vi "GeoData.vi"() -> ()   [LabVIEW 2017] (continued)
UT\tCache County\tH1\n84318\t49005\tHyde park\tUT\tCache County\tH1\n84338\t49005\tTrenton\tUT\tCache County\tH1\n84332\t49005\tProvidence\tUT\tCache County\tH1\n84305\t49005\tClarkston\tUT\tCache County\tH1\n84312\t49005\tGarland\tUT\tCache County\tH1\n84328\t49005\tParadise\tUT\tCache County\tH1\n84341\t49005\tLogan\tUT\tCache County\tH1\n84322\t49005\tLogan\tUT\tCache County\tH1\n84319\t49005\tHyrum\tUT\tCache County\tH1\n84325\t49005\tMendon\tUT\tCache County\tH1\n84320\t49005\tLewiston\tUT\tCache County\tH1\n84501\t49007\tPrice\tUT\tCarbon County\tH1\n84529\t49007\tKenilworth\tUT\tCarbon County\tH1\n84542\t49007\tWellington\tUT\tCarbon County\tH1\n84526\t49007\tHelper\tUT\tCarbon County\tH1\n84520\t49007\tEast carbon\tUT\tCarbon County\tH1\n84539\t49007\tSunnyside\tUT\tCarbon County\tH1\n84046\t49009\tManila\tUT\tDaggett County\tH1\n84023\t49009\tDutch john\tUT\tDaggett County\tH1\n84054\t49011\tNorth salt lake\tUT\tDavis County\tH1\n84315\t49011\tHooper\tUT\tDavis County\tH1\n84011\t49011\tBountiful\tUT\tDavis County\tH1\n84075\t49011\tSyracuse\tUT\tDavis County\tH1\n84041\t49011\tLayton\tUT\tDavis County\tH1\n84037\t49011\tKaysville\tUT\tDavis County\tH1\n84405\t49011\tOgden\tUT\tDavis County\tH1\n84025\t49011\tFarmington\tUT\tDavis County\tH1\n84014\t49011\tCenterville\tUT\tDavis County\tH1\n84015\t49011\tClearfield\tUT\tDavis County\tH1\n84087\t49011\tWoods cross\tUT\tDavis County\tH1\n84016\t49011\tClearfield\tUT\tDavis County\tH1\n84089\t49011\tClearfield\tUT\tDavis County\tH1\n84010\t49011\tBountiful\tUT\tDavis County\tH1\n84040\t49011\tLayton\tUT\tDavis County\tH1\n84056\t49011\tHill afb\tUT\tDavis County\tH1\n84031\t49013\tHanna\tUT\tDuchesne County\tH1\n84066\t49013\tRoosevelt\tUT\tDuchesne County\tH1\n84072\t49013\tTabiona\tUT\tDuchesne County\tH1\n84073\t49013\tTalmage\tUT\tDuchesne County\tH1\n84052\t49013\tMyton\tUT\tDuchesne County\tH1\n84021\t49013\tDuchesne\tUT\tDuchesne County\tH1\n84051\t49013\tMountain home\tUT\tDuchesne County\tH1\n84007\t49013\tBluebell\tUT\tDuchesne County\tH1\n84053\t49013\tNeola\tUT\tDuchesne County\tH1\n84001\t49013\tAltamont\tUT\tDuchesne County\tH1\n84002\t49013\tAltonah\tUT\tDuchesne County\tH1\n84027\t49013\tFruitland\tUT\tDuchesne County\tH1\n84501\t49015\tPrice\tUT\tEmery County\tH1\n84521\t49015\tElmo\tUT\tEmery County\tH1\n84523\t49015\tFerron\tUT\tEmery County\tH1\n84537\t49015\tOrangeville\tUT\tEmery County\tH1\n84522\t49015\tEmery\tUT\tEmery County\tH1\n84518\t49015\tCleveland\tUT\tEmery County\tH1\n84528\t49015\tHuntington\tUT\tEmery County\tH1\n84525\t49015\tGreen river\tUT\tEmery County\tH1\n84516\t49015\tClawson\tUT\tEmery County\tH1\n84513\t49015\tCastle dale\tUT\tEmery County\tH1\n84716\t49017\tBoulder\tUT\tGarfield County\tH1\n84718\t49017\tCannonville\tUT\tGarfield County\tH1\n84764\t49017\tBryce\tUT\tGarfield County\tH1\n84736\t49017\tHenrieville\tUT\tGarfield County\tH1\n84712\t49017\tAntimony\tUT\tGarfield County\tH1\n84726\t49017\tEscalante\tUT\tGarfield County\tH1\n84759\t49017\tPanguitch\tUT\tGarfield County\tH1\n84776\t49017\tTropic\tUT\tGarfield County\tH1\n84515\t49019\tCisco\tUT\tGrand County\tH1\n84525\t49019\tGreen river\tUT\tGrand County\tH1\n84532\t49019\tMoab\tUT\tGrand County\tH1\n84540\t49019\tThompson\tUT\tGrand County\tH1\n84781\t49021\tPine valley\tUT\tIron County\tH1\n84722\t49021\tCentral\tUT\tIron County\tH1\n84761\t49021\tParowan\tUT\tIron County\tH1\n84721\t49021\tCedar city\tUT\tIron County\tH1\n84720\t49021\tCedar city\tUT\tIron County\tH1\n84742\t49021\tKanarraville\tUT\tIron County\tH1\n84757\t49021\tNew harmony\tUT\tIron County\tH1\n84714\t49021\tBeryl\tUT\tIron County\tH1\n84753\t49021\tModena\tUT\tIron County\tH1\n84719\t49021\tBrian head\tUT\tIron County\tH1\n84756\t49021\tNewcastle\tUT\tIron County\tH1\n84760\t49021\tParagonah\tUT\tIron County\tH1\n84737\t49021\tHurricane\tUT\tIron County\tH1\n84772\t49021\tSummit\tUT\tIron County\tH1\n84639\t49023\tLevan\tUT\tJuab County\tH1\n84628\t49023\tEureka\tUT\tJuab County\tH1\n84648\t49023\tNephi\tUT\tJuab County\tH1\n84645\t49023\tMona\tUT\tJuab County\tH1\n84758\t49025\tOrderville\tUT\tKane County\tH1\n84735\t49025\tHatch\tUT\tKane County\tH1\n84729\t49025\tGlendale\tUT\tKane County\tH1\n84710\t49025\tAlton\tUT\tKane County\tH1\n84726\t49025\tEscalante\tUT\tKane County\tH1\n84762\t49025\tDuck creek village\tUT\tKane County\tH1\n84755\t49025\tMount carmel\tUT\tKane County\tH1\n84741\t49025\tKanab\tUT\tKane County\tH1\n84635\t49027\tHinckley\tUT\tMillard County\tH1\n84656\t49027\tScipio\tUT\tMillard County\tH1\n84631\t49027\tFillmore\tUT\tMillard County\tH1\n84640\t49027\tLynndyl\tUT\tMillard County\tH1\n84728\t49027\tGarrison\tUT\tMillard County\tH1\n84649\t49027\tOak city\tUT\tMillard County\tH1\n84638\t49027\tLeamington\tUT\tMillard County\tH1\n84637\t49027\tKanosh\tUT\tMillard County\tH1\n84624\t49027\tDelta\tUT\tMillard County\tH1\n84636\t49027\tHolden\tUT\tMillard County\tH1\n84644\t49027\tMeadow\tUT\tMillard County\tH1\n84018\t49029\tCroydon\tUT\tMorgan County\tH1\n84050\t49029\tMorgan\tUT\tMorgan County\tH1\n84017\t49029\tCoalville\tUT\tMorgan County\tH1\n84750\t49031\tMarysvale\tUT\tPiute County\tH1\n84743\t49031\tKingston\tUT\tPiute County\tH1\n84712\t49031\tAntimony\tUT\tPiute County\tH1\n84732\t49031\tGreenwich\tUT\tPiute County\tH1\n84723\t49031\tCircleville\tUT\tPiute County\tH1\n84740\t49031\tJunction\tUT\tPiute County\tH1\n84064\t49033\tRandolph\tUT\tRich County\tH1\n84086\t49033\tWoodruff\tUT\tRich County\tH1\n84038\t49033\tLaketown\tUT\tRich County\tH1\n84028\t49033\tGarden city\tUT\tRich County\tH1\n84070\t49035\tSandy\tUT\tSalt Lake County\tH1\n84123\t49035\tSalt lake city\tUT\tSalt Lake County\tH1\n84129\t49035\tSalt lake city\tUT\tSalt Lake County\tH1\n84152\t49035\tSalt lake city\tUT\tSalt Lake County\tH1\n84101\t49035\tSalt lake city\tUT\tSalt Lake County\tH1\n84103\t49035\tSalt lake city\tUT\tSalt Lake County\tH1\n84118\t49035\tSalt lake city\tUT\tSalt Lake County\tH1\n84127\t49035\tSalt lake city\tUT\tSalt Lake County\tH1\n84134\t49035\tSalt lake city\tUT\tSalt Lake County\tH1\n84184\t49035\tSalt lake city\tUT\tSalt Lake County\tH1\n84119\t49035\tWest valley city\tUT\tSalt Lake County\tH1\n84138\t49035\tSalt lake city\tUT\tSalt Lake County\tH1\n84143\t49035\tSalt lake city\tUT\tSalt Lake County\tH1\n84047\t49035\tMidvale\tUT\tSalt Lake County\tH1\n84050\t49035\tMorgan\tUT\tSalt Lake County\tH1\n84107\t49035\tSalt lake city\tUT\tSalt Lake County\tH1\n84092\t49035\tSandy\tUT\tSalt Lake County\tH1\n84158\t49035\tSalt lake city\tUT\tSalt Lake County\tH1\n84112\t49035\tSalt lake city\tUT\tSalt Lake County\tH1\n84132\t49035\tSalt lake city\tUT\tSalt Lake County\tH1\n84009\t49035\tSouth jordan\tUT\tSalt Lake County\tH1\n84065\t49035\tRiverton\tUT\tSalt Lake County\tH1\n84084\t49035\tWest jordan\tUT\tSalt Lake County\tH1\n84102\t49035\tSalt lake city\tUT\tSalt Lake County\tH1\n84106\t49035\tSalt lake city\tUT\tSalt Lake County\tH1\n84115\t49035\tSalt lake city\tUT\tSalt Lake County\tH1\n84090\t49035\tSandy\tUT\tSalt Lake County\tH1\n84096\t49035\tHerriman\tUT\tSalt Lake County\tH1\n84088\t49035\tWest jordan\tUT\tSalt Lake County\tH1\n84105\t49035\tSalt lake city\tUT\tSalt Lake County\tH1\n84150\t49035\tSalt lake city\tUT\tSalt Lake County\tH1\n84122\t49035\tSalt lake city\tUT\tSalt Lake County\tH1\n84141\t49035\tSalt lake city\tUT\tSalt Lake County\tH1\n84139\t49035\tSalt lake city\tUT\tSalt Lake County\tH1\n84020\t49035\tDraper\tUT\tSalt Lake County\tH1\n84157\t49035\tSalt lake city\tUT\tSalt Lake County\tH1\n84104\t49035\tSalt lake city\tUT\tSalt Lake County\tH1\n84120\t49035\tWest valley city\tUT\tSalt Lake County\tH1\n84121\t49035\tSalt lake city\tUT\tSalt Lake County\tH1\n84133\t49035\tSalt lake city\tUT\tSalt Lake County\tH1\n84113\t49035\tSalt lake city\tUT\tSalt Lake County\tH1\n84148\t49035\tSalt lake city\tUT\tSalt Lake County\tH1\n84128\t49035\tWest valley city\tUT\tSalt Lake County\tH1\n84108\t49035\tSalt lake city\tUT\tSalt Lake County\tH1\n84117\t49035\tSalt lake city\tUT\tSalt Lake County\tH1\n84095\t49035\tSouth jordan\tUT\tSalt Lake County\tH1\n84093\t49035\tSandy\tUT\tSalt Lake County\tH1\n84126\t49035\tSalt lake city\tUT\tSalt Lake County\tH1\n84165\t49035\tSalt lake city\tUT\tSalt Lake County\tH1\n84171\t49035\tSalt lake city\tUT\tSalt Lake County\tH1\n84110\t49035\tSalt lake city\tUT\tSalt Lake County\tH1\n84091\t49035\tSandy\tUT\tSalt Lake County\tH1\n84199\t49035\tSalt lake city\tUT\tSalt Lake County\tH1\n84190\t49035\tSalt lake city\tUT\tSalt Lake County\tH1\n84151\t49035\tSalt lake city\tUT\tSalt Lake County\tH1\n84124\t49035\tSalt lake city\tUT\tSalt Lake County\tH1\n84109\t49035\tSalt lake city\tUT\tSalt Lake County\tH1\n84094\t49035\tSandy\tUT\tSalt Lake County\tH1\n84116\t49035\tSalt lake city\tUT\tSalt Lake County\tH1\n84125\t49035\tSalt lake city\tUT\tSalt Lake County\tH1\n84044\t49035\tMagna\tUT\tSalt Lake County\tH1\n84081\t49035\tWest jordan\tUT\tSalt Lake County\tH1\n84111\t49035\tSalt lake city\tUT\tSalt Lake County\tH1\n84180\t49035\tSalt lake city\tUT\tSalt Lake County\tH1\n84006\t49035\tBingham canyon\tUT\tSalt Lake County\tH1\n84170\t49035\tSalt lake city\tUT\tSalt Lake County\tH1\n84114\t49035\tSalt lake city\tUT\tSalt Lake County\tH1\n84533\t49037\tLake powell\tUT\tSan Juan County\tH1\n84512\t49037\tBluff\tUT\tSan Juan County\tH1\n84511\t49037\tBlanding\tUT\tSan Juan County\tH1\n84535\t49037\tMonticello\tUT\tSan Juan County\tH1\n84531\t49037\tMexican hat\tUT\tSan Juan County\tH1\n84532\t49037\tMoab\tUT\tSan Juan County\tH1\n84510\t49037\tAneth\tUT\tSan Juan County\tH1\n84530\t49037\tLa sal\tUT\tSan Juan County\tH1\n84534\t49037\tMontezuma creek\tUT\tSan Juan County\tH1\n84536\t49037\tMonument valley\tUT\tSan Juan County\tH1\n84629\t49039\tFairview\tUT\tSanpete County\tH1\n84622\t49039\tCenterfield\tUT\tSanpete County\tH1\n84630\t49039\tFayette\tUT\tSanpete County\tH1\n84665\t49039\tSterling\tUT\tSanpete County\tH1\n84647\t49039\tMount pleasant\tUT\tSanpete County\tH1\n84627\t49039\tEphraim\tUT\tSanpete County\tH1\n84642\t49039\tManti\tUT\tSanpete County\tH1\n84667\t49039\tWales\tUT\tSanpete County\tH1\n84643\t49039\tMayfield\tUT\tSanpete County\tH1\n84634\t49039\tGunnison\tUT\tSanpete County\tH1\n84632\t49039\tFountain green\tUT\tSanpete County\tH1\n84621\t49039\tAxtell\tUT\tSanpete County\tH1\n84662\t49039\tSpring city\tUT\tSanpete County\tH1\n84646\t49039\tMoroni\tUT\tSanpete County\tH1\n84623\t49039\tChester\tUT\tSanpete County\tH1\n84739\t49041\tJoseph\tUT\tSevier County\tH1\n84754\t49041\tMonroe\tUT\tSevier County\tH1\n84654\t49041\tSalina\tUT\tSevier County\tH1\n84620\t49041\tAurora\tUT\tSevier County\tH1\n84744\t49041\tKoosharem\tUT\tSevier County\tH1\n84711\t49041\tAnnabella\tUT\tSevier County\tH1\n84730\t49041\tGlenwood\tUT\tSevier County\tH1\n84657\t49041\tSigurd\tUT\tSevier County\tH1\n84701\t49041\tRichfield\tUT\tSevier County\tH1\n84766\t49041\tSevier\tUT\tSevier County\tH1\n84652\t49041\tRedmond\tUT\tSevier County\tH1\n84724\t49041\tElsinore\tUT\tSevier County\tH1\n84033\t49043\tHenefer\tUT\tSummit County\tH1\n84024\t49043\tEcho\tUT\tSummit County\tH1\n84055\t49043\tOakley\tUT\tSummit County\tH1\n84060\t49043\tPark city\tUT\tSummit County\tH1\n84017\t49043\tCoalville\tUT\tSummit County\tH1\n84036\t49043\tKamas\tUT\tSummit County\tH1\n84068\t49043\tPark city\tUT\tSummit County\tH1\n84098\t49043\tPark city\tUT\tSummit County\tH1\n84061\t49043\tPeoa\tUT\tSummit County\tH1\n84074\t49045\tTooele\tUT\tTooele County\tH1\n84029\t49045\tGrantsville\tUT\tTooele County\tH1\n84034\t49045\tIbapah\tUT\tTooele County\tH1\n84083\t49045\tWendover\tUT\tTooele County\tH1\n84069\t49045\tRush valley\tUT\tTooele County\tH1\n84071\t49045\tStockton\tUT\tTooele County\tH1\n84022\t49045\tDugway\tUT\tTooele County\tH1\n84080\t49045\tVernon\tUT\tTooele County\tH1\n84079\t49047\tVernal\tUT\tUintah County\tH1\n84066\t49047\tRoosevelt\tUT\tUintah County\tH1\n84035\t49047\tJensen\tUT\tUintah County\tH1\n84063\t49047\tRandlett\tUT\tUintah County\tH1\n84078\t49047\tVernal\tUT\tUintah County\tH1\n84039\t49047\tLapoint\tUT\tUintah County\tH1\n84026\t49047\tFort duchesne\tUT\tUintah County\tH1\n84085\t49047\tWhiterocks\tUT\tUintah County\tH1\n84076\t49047\tTridell\tUT\tUintah County\tH1\n84008\t49047\tBonanza\tUT\tUintah County\tH1\n84043\t49049\tLehi\tUT\tUtah County\tH1\n84059\t49049\tOrem\tUT\tUtah County\tH1\n84004\t49049\tAlpine\tUT\tUtah County\tH1\n84097\t49049\tOrem\tUT\tUtah County\tH1\n84013\t49049\tCedar valley\tUT\tUtah County\tH1\n84603\t49049\tProvo\tUT\tUtah County\tH1\n84604\t49049\tProvo\tUT\tUtah County\tH1\n84655\t49049\tSantaquin\tUT\tUtah County\tH1\n84032\t49049\tHeber city\tUT\tUtah County\tH1\n84602\t49049\tProvo\tUT\tUtah County\tH1\n84005\t49049\tEagle mountain\tUT\tUtah County\tH1\n84020\t49049\tDraper\tUT\tUtah County\tH1\n84062\t49049\tPleasant grove\tUT\tUtah County\tH1\n84058\t49049\tOrem\tUT\tUtah County\tH1\n84660\t49049\tSpanish fork\tUT\tUtah County\tH1\n84606\t49049\tProvo\tUT\tUtah County\tH1\n84003\t49049\tAmerican fork\tUT\tUtah County\tH1\n84601\t49049\tProvo\tUT\tUtah County\tH1\n84651\t49049\tPayson\tUT\tUtah County\tH1\n84605\t49049\tProvo\tUT\tUtah County\tH1\n84626\t49049\tElberta\tUT\tUtah County\tH1\n84057\t49049\tOrem\tUT\tUtah County\tH1\n84045\t49049\tSaratoga springs\tUT\tUtah County\tH1\n84042\t49049\tLindon\tUT\tUtah County\tH1\n84663\t49049\tSpringville\tUT\tUtah County\tH1\n84653\t49049\tSalem\tUT\tUtah County\tH1\n84664\t49049\tMapleton\tUT\tUtah County\tH1\n84633\t49049\tGoshen\tUT\tUtah County\tH1\n84604\t49051\tProvo\tUT\tWasatch County\tH1\n84082\t49051\tWallsburg\tUT\tWasatch County\tH1\n84032\t49051\tHeber city\tUT\tWasatch County\tH1\n84060\t49051\tPark city\tUT\tWasatch County\tH1\n84036\t49051\tKamas\tUT\tWasatch County\tH1\n84049\t49051\tMidway\tUT\tWasatch County\tH1\n84779\t49053\tVirgin\tUT\tWashington County\tH1\n84781\t49053\tPine valley\tUT\tWashington County\tH1\n84763\t49053\tRockville\tUT\tWashington County\tH1\n84722\t49053\tCentral\tUT\tWashington County\tH1\n84733\t49053\tGunlock\tUT\tWashington County\tH1\n84782\t49053\tVeyo\tUT\tWashington County\tH1\n84784\t49053\tHildale\tUT\tWashington County\tH1\n84780\t49053\tWashington\tUT\tWashington County\tH1\n84791\t49053\tSaint george\tUT\tWashington County\tH1\n84720\t49053\tCedar city\tUT\tWashington County\tH1\n84765\t49053\tSanta clara\tUT\tWashington County\tH1\n84771\t49053\tSaint george\tUT\tWashington County\tH1\n84783\t49053\tDammeron valley\tUT\tWashington County\tH1\n84757\t49053\tNew harmony\tUT\tWashington County\tH1\n84790\t49053\tSaint george\tUT\tWashington County\tH1\n84745\t49053\tLa verkin\tUT\tWashington County\tH1\n84746\t49053\tLeeds\tUT\tWashington County\tH1\n84738\t49053\tIvins\tUT\tWashington County\tH1\n84774\t49053\tToquerville\tUT\tWashington County\tH1\n84767\t49053\tSpringdale\tUT\tWashington County\tH1\n84725\t49053\tEnterprise\tUT\tWashington County\tH1\n84770\t49053\tSaint george\tUT\tWashington County\tH1\n84737\t49053\tHurricane\tUT\tWashington County\tH1\n84715\t49055\tBicknell\tUT\tWayne County\tH1\n84734\t49055\tHanksville\tUT\tWayne County\tH1\n84747\t49055\tLoa\tUT\tWayne County\tH1\n84775\t49055\tTorrey\tUT\tWayne County\tH1\n84749\t49055\tLyman\tUT\tWayne County\tH1\n84773\t49055\tTeasdale\tUT\tWayne County\tH1\n84310\t49057\tEden\tUT\tWeber County\tH1\n84315\t49057\tHooper\tUT\tWeber County\tH1\n84407\t49057\tOgden\tUT\tWeber County\tH1\n84409\t49057\tOgden\tUT\tWeber County\tH1\n84201\t49057\tOgden\tUT\tWeber County\tH1\n84404\t49057\tOgden\tUT\tWeber County\tH1\n84405\t49057\tOgden\tUT\tWeber County\tH1\n84317\t49057\tHuntsville\tUT\tWeber County\tH1\n84415\t49057\tOgden\tUT\tWeber County\tH1\n84403\t49057\tOgden\tUT\tWeber County\tH1\n84414\t49057\tOgden\tUT\tWeber County\tH1\n84408\t49057\tOgden\tUT\tWeber County\tH1\n84402\t49057\tOgden\tUT\tWeber County\tH1\n84401\t49057\tOgden\tUT\tWeber County\tH1\n84067\t49057\tRoy\tUT\tWeber County\tH1\n84056\t49057\tHill afb\tUT\tWeber County\tH1\n84412\t49057\tOgden\tUT\tWeber County\tH1\n5733\t50001\tBrandon\tVT\tAddison County\tH1\n5747\t50001\tGranville\tVT\tAddison County\tH1\n5753\t50001\tMiddlebury\tVT\tAddison County\tH1\n5472\t50001\tNew haven\tVT\tAddison County\tH1\n5769\t50001\tSalisbury\tVT\tAddison County\tH1\n5469\t50001\tMonkton\tVT\tAddison County\tH1\n5748\t50001\tHancock\tVT\tAddison County\tH1\n5734\t50001\tBridport\tVT\tAddison County\tH1\n5770\t50001\tShoreham\tVT\tAddison County\tH1\n5766\t50001\tRipton\tVT\tAddison County\tH1\n5443\t50001\tBristol\tVT\tAddison County\tH1\n5456\t50001\tFerrisburgh\tVT\tAddison County\tH1\n5491\t50001\tVergennes\tVT\tAddison County\tH1\n5669\t50001\tRoxbury\tVT\tAddison County\tH1\n5740\t50001\tEast middlebury\tVT\tAddison County\tH1\n5461\t50001\tHinesburg\tVT\tAddison County\tH1\n5473\t50001\tNorth ferrisburgh\tVT\tAddison County\tH1\n5462\t50001\tHuntington\tVT\tAddison County\tH1\n5445\t50001\tCharlotte\tVT\tAddison County\tH1\n5487\t50001\tStarksboro\tVT\tAddison County\tH1\n5767\t50001\tRochester\tVT\tAddison County\tH1\n5760\t50001\tOrwell\tVT\tAddison County\tH1\n5778\t50001\tWhiting\tVT\tAddison County\tH1\n5255\t50003\tManchester center\tVT\tBennington County\tH1\n5340\t50003\tBondville\tVT\tBennington County\tH1\n5148\t50003\tLondonderry\tVT\tBennington County\tH1\n5261\t50003\tPownal\tVT\tBennington County\tH1\n5352\t50003\tStamford\tVT\tBennington County\tH1\n5343\t50003\tJamaica\tVT\tBennington County\tH1\n5775\t50003\tWest pawlet\tVT\tBennington County\tH1\n5155\t50003\tSouth londonderry\tVT\tBennington County\tH1\n5201\t50003\tBennington\tVT\tBennington County\tH1\n5250\t50003\tArlington\tVT\tBennington County\tH1\n5257\t50003\tNorth bennington\tVT\tBennington County\tH1\n5761\t50003\tPawlet\tVT\tBennington County\tH1\n5152\t50003\tPeru\tVT\tBennington County\tH1\n5252\t50003\tEast arlington\tVT\tBennington County\tH1\n5253\t50003\tEast dorset\tVT\tBennington County\tH1\n5262\t50003\tShaftsbury\tVT\tBennington County\tH1\n5254\t50003\tManchester\tVT\tBennington County\tH1\n5251\t50003\tDorset\tVT\tBennington County\tH1\n5768\t50003\tRupert\tVT\tBennington County\tH1\n5260\t50003\tNorth pownal\tVT\tBennington County\tH1\n5161\t50003\tWeston\tVT\tBennington County\tH1\n5363\t50003\tWilmington\tVT\tBennington County\tH1\n5350\t50003\tReadsboro\tVT\tBennington County\tH1\n5776\t50003\tWest rupert\tVT\tBennington County\tH1\n5680\t50005\tWolcott\tVT\tCaledonia County\tH1\n5839\t50005\tGlover\tVT\tCaledonia County\tH1\n5849\t50005\tLyndon\tVT\tCaledonia County\tH1\n5861\t50005\tPassumpsic\tVT\tCaledonia County\tH1\n5821\t50005\tBarnet\tVT\tCaledonia County\tH1\n5850\t50005\tLyndon center\tVT\tCaledonia County\tH1\n5832\t50005\tEast burke\tVT\tCaledonia County\tH1\n5873\t50005\tWest danville\tVT\tCaledonia County\tH1\n5647\t50005\tCabot\tVT\tCaledonia County\tH1\n5819\t50005\tSaint johnsbury\tVT\tCaledonia County\tH1\n5866\t50005\tSheffield\tVT\tCaledonia County\tH1\n5871\t50005\tWest burke\tVT\tCaledonia County\tH1\n5838\t50005\tEast saint johnsbury\tVT\tCaledonia County\tH1\n5081\t50005\tWells river\tVT\tCaledonia County\tH1\n5046\t50005\tGroton\tVT\tCaledonia County\tH1\n5836\t50005\tEast hardwick\tVT\tCaledonia County\tH1\n5837\t50005\tEast haven\tVT\tCaledonia County\tH1\n5862\t50005\tPeacham\tVT\tCaledonia County\tH1\n5828\t50005\tDanville\tVT\tCaledonia County\tH1\n5824\t50005\tConcord\tVT\tCaledonia County\tH1\n5867\t50005\tSutton\tVT\tCaledonia County\tH1\n5863\t50005\tSaint johnsbury center\tVT\tCaledonia County\tH1\n5842\t50005\tGreensboro bend\tVT\tCaledonia County\tH1\n5050\t50005\tMc indoe falls\tVT\tCaledonia County\tH1\n5069\t50005\tSouth ryegate\tVT\tCaledonia County\tH1\n5658\t50005\tMarshfield\tVT\tCaledonia County\tH1\n5841\t50005\tGreensboro\tVT\tCaledonia County\tH1\n5851\t50005\tLyndonville\tVT\tCaledonia County\tH1\n5843\t50005\tHardwick\tVT\tCaledonia County\tH1\n5042\t50005\tEast ryegate\tVT\tCaledonia County\tH1\n5848\t50005\tLower waterford\tVT\tCaledonia County\tH1\n5403\t50007\tSouth burlington\tVT\tChittenden County\tH1\n5446\t50007\tColchester\tVT\tChittenden County\tH1\n5449\t50007\tColchester\tVT\tChittenden County\tH1\n5676\t50007\tWaterbury\tVT\tChittenden County\tH1\n5490\t50007\tUnderhill center\tVT\tChittenden County\tH1\n5495\t50007\tWilliston\tVT\tChittenden County\tH1\n5401\t50007\tBurlington\tVT\tChittenden County\tH1\n5452\t50007\tEssex junction\tVT\tChittenden County\tH1\n5482\t50007\tShelburne\tVT\tChittenden County\tH1\n5406\t50007\tBurlington\tVT\tChittenden County\tH1\n5466\t50007\tJonesville\tVT\tChittenden County\tH1\n5402\t50007\tBurlington\tVT\tChittenden County\tH1\n5477\t50007\tRichmond\tVT\tChittenden County\tH1\n5465\t50007\tJericho\tVT\tChittenden County\tH1\n5453\t50007\tEssex junction\tVT\tChittenden County\tH1\n5451\t50007\tEssex\tVT\tChittenden County\tH1\n5439\t50007\tColchester\tVT\tChittenden County\tH1\n5408\t50007\tBurlington\tVT\tChittenden County\tH1\n5489\t50007\tUnderhill\tVT\tChittenden County\tH1\n5404\t50007\tWinooski\tVT\tChittenden County\tH1\n5468\t50007\tMilton\tVT\tChittenden County\tH1\n5478\t50007\tSaint albans\tVT\tChittenden County\tH1\n5454\t50007\tFairfax\tVT\tChittenden County\tH1\n5461\t50007\tHinesburg\tVT\tChittenden County\tH1\n5473\t50007\tNorth ferrisburgh\tVT\tChittenden County\tH1\n5462\t50007\tHuntington\tVT\tChittenden County\tH1\n5445\t50007\tCharlotte\tVT\tChittenden County\tH1\n5487\t50007\tStarksboro\tVT\tChittenden County\tH1\n5405\t50007\tBurlington\tVT\tChittenden County\tH1\n5494\t50007\tWestford\tVT\tChittenden County\tH1\n5407\t50007\tSouth burlington\tVT\tChittenden County\tH1\n5858\t50009\tNorth concord\tVT\tEssex County\tH1\n5905\t50009\tGuildhall\tVT\tEssex County\tH1\n5907\t50009\tNorton\tVT\tEssex County\tH1\n5906\t50009\tLunenburg\tVT\tEssex County\tH1\n5902\t50009\tBeecher falls\tVT\tEssex County\tH1\n5819\t50009\tSaint johnsbury\tVT\tEssex County\tH1\n5871\t50009\tWest burke\tVT\tEssex County\tH1\n5846\t50009\tIsland pond\tVT\tEssex County\tH1\n5903\t50009\tCanaan\tVT\tEssex County\tH1\n5837\t50009\tEast haven\tVT\tEssex County\tH1\n5840\t50009\tGranby\tVT\tEssex County\tH1\n5824\t50009\tConcord\tVT\tEssex County\tH1\n5901\t50009\tAverill\tVT\tEssex County\tH1\n5904\t50009\tGilman\tVT\tEssex County\tH1\n5450\t50011\tEnosburg falls\tVT\tFranklin County\tH1\n5859\t50011\tNorth troy\tVT\tFranklin County\tH1\n5485\t50011\tSheldon springs\tVT\tFranklin County\tH1\n5481\t50011\tSaint albans bay\tVT\tFranklin County\tH1\n5460\t50011\tHighgate springs\tVT\tFranklin County\tH1\n5488\t50011\tSwanton\tVT\tFranklin County\tH1\n5476\t50011\tRichford\tVT\tFranklin County\tH1\n5441\t50011\tBakersfield\tVT\tFranklin County\tH1\n5479\t50011\tSaint albans\tVT\tFranklin County\tH1\n5448\t50011\tEast fairfield\tVT\tFranklin County\tH1\n5459\t50011\tHighgate center\tVT\tFranklin County\tH1\n5468\t50011\tMilton\tVT\tFranklin County\tH1\n5478\t50011\tSaint albans\tVT\tFranklin County\tH1\n5455\t50011\tFairfield\tVT\tFranklin County\tH1\n5454\t50011\tFairfax\tVT\tFranklin County\tH1\n5457\t50011\tFranklin\tVT\tFranklin County\tH1\n5464\t50011\tJeffersonville\tVT\tFranklin County\tH1\n5444\t50011\tCambridge\tVT\tFranklin County\tH1\n5483\t50011\tSheldon\tVT\tFranklin County\tH1\n5471\t50011\tMontgomery center\tVT\tFranklin County\tH1\n5447\t50011\tEast berkshire\tVT\tFranklin County\tH1\n5470\t50011\tMontgomery\tVT\tFranklin County\tH1\n5486\t50013\tSouth hero\tVT\tGrand Isle County\tH1\n5474\t50013\tNorth hero\tVT\tGrand Isle County\tH1\n5458\t50013\tGrand isle\tVT\tGrand Isle County\tH1\n5463\t50013\tIsle la motte\tVT\tGrand Isle County\tH1\n5440\t50013\tAlburgh\tVT\tGrand Isle County\tH1\n5442\t50015\tBelvidere center\tVT\tLamoille County\tH1\n5661\t50015\tMorrisville\tVT\tLamoille County\tH1\n5680\t50015\tWolcott\tVT\tLamoille County\tH1\n5652\t50015\tEden\tVT\tLamoille County\tH1\n5665\t50015\tNorth hyde park\tVT\tLamoille County\tH1\n5492\t50015\tWaterville\tVT\tLamoille County\tH1\n5655\t50015\tHyde park\tVT\tLamoille County\tH1\n5826\t50015\tCraftsbury\tVT\tLamoille County\tH1\n5653\t50015\tEden mills\tVT\tLamoille County\tH1\n5489\t50015\tUnderhill\tVT\tLamoille County\tH1\n5657\t50015\tLake elmore\tVT\tLamoille County\tH1\n5464\t50015\tJeffersonville\tVT\tLamoille County\tH1\n5444\t50015\tCambridge\tVT\tLamoille County\tH1\n5656\t50015\tJohnson\tVT\tLamoille County\tH1\n5672\t50015\tStowe\tVT\tLamoille County\tH1\n5843\t50015\tHardwick\tVT\tLamoille County\tH1\n5662\t50015\tMoscow\tVT\tLamoille County\tH1\n5061\t50017\tRandolph center\tVT\tOrange County\tH1\n5079\t50017\tVershire\tVT\tOrange County\tH1\n5641\t50017\tBarre\tVT\tOrange County\tH1\n5055\t50017\tNorwich\tVT\tOrange County\tH1\n5045\t50017\tFairlee\tVT\tOrange County\tH1\n5033\t50017\tBradford\tVT\tOrange County\tH1\n5663\t50017\tNorthfield\tVT\tOrange County\tH1\n5072\t50017\tStrafford\tVT\tOrange County\tH1\n5076\t50017\tTopsham\tVT\tOrange County\tH1\n5032\t50017\tBethel\tVT\tOrange County\tH1\n5086\t50017\tWest topsham\tVT\tOrange County\tH1\n5054\t50017\tNorth thetford\tVT\tOrange County\tH1\n5085\t50017\tWest newbury\tVT\tOrange County\tH1\n5043\t50017\tEast thetford\tVT\tOrange County\tH1\n5038\t50017\tChelsea\tVT\tOrange County\tH1\n5041\t50017\tEast randolph\tVT\tOrange County\tH1\n5060\t50017\tRandolph\tVT\tOrange County\tH1\n5654\t50017\tGraniteville\tVT\tOrange County\tH1\n5070\t50017\tSouth strafford\tVT\tOrange County\tH1\n5051\t50017\tNewbury\tVT\tOrange County\tH1\n5081\t50017\tWells river\tVT\tOrange County\tH1\n5046\t50017\tGroton\tVT\tOrange County\tH1\n5036\t50017\tBrookfield\tVT\tOrange County\tH1\n5679\t50017\tWilliamstown\tVT\tOrange County\tH1\n5675\t50017\tWashington\tVT\tOrange County\tH1\n5039\t50017\tCorinth\tVT\tOrange County\tH1\n5649\t50017\tEast barre\tVT\tOrange County\tH1\n5065\t50017\tSharon\tVT\tOrange County\tH1\n5068\t50017\tSouth royalton\tVT\tOrange County\tH1\n5669\t50017\tRoxbury\tVT\tOrange County\tH1\n5083\t50017\tWest fairlee\tVT\tOrange County\tH1\n5074\t50017\tThetford\tVT\tOrange County\tH1\n5077\t50017\tTunbridge\tVT\tOrange County\tH1\n5069\t50017\tSouth ryegate\tVT\tOrange County\tH1\n5075\t50017\tThetford center\tVT\tOrange County\tH1\n5040\t50017\tEast corinth\tVT\tOrange County\tH1\n5058\t50017\tPost mills\tVT\tOrange County\tH1\n5680\t50019\tWolcott\tVT\tOrleans County\tH1\n5859\t50019\tNorth troy\tVT\tOrleans County\tH1\n5827\t50019\tCraftsbury common\tVT\tOrleans County\tH1\n5839\t50019\tGlover\tVT\tOrleans County\tH1\n5825\t50019\tCoventry\tVT\tOrleans County\tH1\n5845\t50019\tIrasburg\tVT\tOrleans County\tH1\n5868\t50019\tTroy\tVT\tOrleans County\tH1\n5847\t50019\tLowell\tVT\tOrleans County\tH1\n5829\t50019\tDerby\tVT\tOrleans County\tH1\n5820\t50019\tAlbany\tVT\tOrleans County\tH1\n5476\t50019\tRichford\tVT\tOrleans County\tH1\n5826\t50019\tCraftsbury\tVT\tOrleans County\tH1\n5872\t50019\tWest charleston\tVT\tOrleans County\tH1\n5871\t50019\tWest burke\tVT\tOrleans County\tH1\n5846\t50019\tIsland pond\tVT\tOrleans County\tH1\n5836\t50019\tEast hardwick\tVT\tOrleans County\tH1\n5857\t50019\tNewport center\tVT\tOrleans County\tH1\n5874\t50019\tWestfield\tVT\tOrleans County\tH1\n5860\t50019\tOrleans\tVT\tOrleans County\tH1\n5823\t50019\tBeebe plain\tVT\tOrleans County\tH1\n5833\t50019\tEast charleston\tVT\tOrleans County\tH1\n5855\t50019\tNewport\tVT\tOrleans County\tH1\n5822\t50019\tBarton\tVT\tOrleans County\tH1\n5830\t50019\tDerby line\tVT\tOrleans County\tH1\n5471\t50019\tMontgomery center\tVT\tOrleans County\tH1\n5842\t50019\tGreensboro bend\tVT\tOrleans County\tH1\n5841\t50019\tGreensboro\tVT\tOrleans County\tH1\n5843\t50019\tHardwick\tVT\tOrleans County\tH1\n5853\t50019\tMorgan\tVT\tOrleans County\tH1\n5875\t50019\tBarton\tVT\tOrleans County\tH1\n5733\t50021\tBrandon\tVT\tRutland County\tH1\n5742\t50021\tEast wallingford\tVT\tRutland County\tH1\n5738\t50021\tCuttingsville\tVT\tRutland County\tH1\n5762\t50021\tPittsfield\tVT\tRutland County\tH1\n5741\t50021\tEast poultney\tVT\tRutland County\tH1\n5701\t50021\tRutland\tVT\tRutland County\tH1\n5730\t50021\tBelmont\tVT\tRutland County\tH1\n5759\t50021\tNorth clarendon\tVT\tRutland County\tH1\n5774\t50021\tWells\tVT\tRutland County\tH1\n5750\t50021\tHydeville\tVT\tRutland County\tH1\n5743\t50021\tFair haven\tVT\tRutland County\tH1\n5763\t50021\tPittsford\tVT\tRutland County\tH1\n5773\t50021\tWallingford\tVT\tRutland County\tH1\n5732\t50021\tBomoseen\tVT\tRutland County\tH1\n5739\t50021\tDanby\tVT\tRutland County\tH1\n5765\t50021\tProctor\tVT\tRutland County\tH1\n5702\t50021\tRutland\tVT\tRutland County\tH1\n5757\t50021\tMiddletown springs\tVT\tRutland County\tH1\n5731\t50021\tBenson\tVT\tRutland County\tH1\n5745\t50021\tForest dale\tVT\tRutland County\tH1\n5737\t50021\tChittenden\tVT\tRutland County\tH1\n5775\t50021\tWest pawlet\tVT\tRutland County\tH1\n5761\t50021\tPawlet\tVT\tRutland County\tH1\n5758\t50021\tMount holly\tVT\tRutland County\tH1\n5772\t50021\tStockbridge\tVT\tRutland County\tH1\n5253\t50021\tEast dorset\tVT\tRutland County\tH1\n5736\t50021\tCenter rutland\tVT\tRutland County\tH1\n5735\t50021\tCastleton\tVT\tRutland County\tH1\n5751\t50021\tKillington\tVT\tRutland County\tH1\n5767\t50021\tRochester\tVT\tRutland County\tH1\n5251\t50021\tDorset\tVT\tRutland County\tH1\n5760\t50021\tOrwell\tVT\tRutland County\tH1\n5744\t50021\tFlorence\tVT\tRutland County\tH1\n5764\t50021\tPoultney\tVT\tRutland County\tH1\n5778\t50021\tWhiting\tVT\tRutland County\tH1\n5777\t50021\tWest rutland\tVT\tRutland County\tH1\n5602\t50023\tMontpelier\tVT\tWashington County\tH1\n5641\t50023\tBarre\tVT\tWashington County\tH1\n5676\t50023\tWaterbury\tVT\tWashington County\tH1\n5667\t50023\tPlainfield\tVT\tWashington County\tH1\n5680\t50023\tWolcott\tVT\tWashington County\tH1\n5671\t50023\tWaterbury\tVT\tWashington County\tH1\n5601\t50023\tMontpelier\tVT\tWashington County\tH1\n5660\t50023\tMoretown\tVT\tWashington County\tH1\n5663\t50023\tNorthfield\tVT\tWashington County\tH1\n5682\t50023\tWorcester\tVT\tWashington County\tH1\n5670\t50023\tSouth barre\tVT\tWashington County\tH1\n5603\t50023\tMontpelier\tVT\tWashington County\tH1\n5674\t50023\tWarren\tVT\tWashington County\tH1\n5873\t50023\tWest danville\tVT\tWashington County\tH1\n5666\t50023\tNorth montpelier\tVT\tWashington County\tH1\n5604\t50023\tMontpelier\tVT\tWashington County\tH1\n5060\t50023\tRandolph\tVT\tWashington County\tH1\n5651\t50023\tEast montpelier\tVT\tWashington County\tH1\n5647\t50023\tCabot\tVT\tWashington County\tH1\n5654\t50023\tGraniteville\tVT\tWashington County\tH1\n5664\t50023\tNorthfield falls\tVT\tWashington County\tH1\n5648\t50023\tCalais\tVT\tWashington County\tH1\n5640\t50023\tAdamant\tVT\tWashington County\tH1\n5609\t50023\tMontpelier\tVT\tWashington County\tH1\n5649\t50023\tEast barre\tVT\tWashington County\tH1\n5669\t50023\tRoxbury\tVT\tWashington County\tH1\n5620\t50023\tMontpelier\tVT\tWashington County\tH1\n5681\t50023\tWoodbury\tVT\tWashington County\tH1\n5650\t50023\tEast calais\tVT\tWashington County\tH1\n5673\t50023\tWaitsfield\tVT\tWashington County\tH1\n5677\t50023\tWaterbury center\tVT\tWashington County\tH1\n5658\t50023\tMarshfield\tVT\tWashington County\tH1\n5633\t50023\tMontpelier\tVT\tWashington County\tH1\n5843\t50023\tHardwick\tVT\tWashington County\tH1\n5678\t50023\tWebsterville\tVT\tWashington County\tH1\n5342\t50025\tJacksonville\tVT\tWindham County\tH1\n5345\t50025\tNewfane\tVT\tWindham County\tH1\n5362\t50025\tWilliamsville\tVT\tWindham County\tH1\n5143\t50025\tChester\tVT\tWindham County\tH1\n5301\t50025\tBrattleboro\tVT\tWindham County\tH1\n5361\t50025\tWhitingham\tVT\tWindham County\tH1\n5358\t50025\tWest halifax\tVT\tWindham County\tH1\n5344\t50025\tMarlboro\tVT\tWindham County\tH1\n5357\t50025\tWest dummerston\tVT\tWindham County\tH1\n5146\t50025\tGrafton\tVT\tWindham County\tH1\n5148\t50025\tLondonderry\tVT\tWindham County\tH1\n5354\t50025\tVernon\tVT\tWindham County\tH1\n5351\t50025\tSouth newfane\tVT\tWindham County\tH1\n5341\t50025\tEast dover\tVT\tWindham County\tH1\n5154\t50025\tSaxtons river\tVT\tWindham County\tH1\n5359\t50025\tWest townshend\tVT\tWindham County\tH1\n5343\t50025\tJamaica\tVT\tWindham County\tH1\n5158\t50025\tWestminster\tVT\tWindham County\tH1\n5355\t50025\tWardsboro\tVT\tWindham County\tH1\n5159\t50025\tWestminster station\tVT\tWindham County\tH1\n5141\t50025\tCambridgeport\tVT\tWindham County\tH1\n5155\t50025\tSouth londonderry\tVT\tWindham County\tH1\n5201\t50025\tBennington\tVT\tWindham County\tH1\n5346\t50025\tPutney\tVT\tWindham County\tH1\n5356\t50025\tWest dover\tVT\tWindham County\tH1\n5156\t50025\tSpringfield\tVT\tWindham County\tH1\n5101\t50025\tBellows falls\tVT\tWindham County\tH1\n5353\t50025\tTownshend\tVT\tWindham County\tH1\n5363\t50025\tWilmington\tVT\tWindham County\tH1\n5350\t50025\tReadsboro\tVT\tWindham County\tH1\n5360\t50025\tWest wardsboro\tVT\tWindham County\tH1\n5089\t50027\tWindsor\tVT\tWindsor County\tH1\n5061\t50027\tRandolph center\tVT\tWindsor County\tH1\n5073\t50027\tTaftsville\tVT\tWindsor County\tH1\n5055\t50027\tNorwich\tVT\tWindsor County\tH1\n5762\t50027\tPittsfield\tVT\tWindsor County\tH1\n5030\t50027\tAscutney\tVT\tWindsor County\tH1\n5150\t50027\tNorth springfield\tVT\tWindsor County\tH1\n5052\t50027\tNorth hartland\tVT\tWindsor County\tH1\n5059\t50027\tQuechee\tVT\tWindsor County\tH1\n5746\t50027\tGaysville\tVT\tWindsor County\tH1\n5143\t50027\tChester\tVT\tWindsor County\tH1\n5149\t50027\tLudlow\tVT\tWindsor County\tH1\n5142\t50027\tCavendish\tVT\tWindsor County\tH1\n5047\t50027\tHartford\tVT\tWindsor County\tH1\n5032\t50027\tBethel\tVT\tWindsor County\tH1\n5148\t50027\tLondonderry\tVT\tWindsor County\tH1\n5153\t50027\tProctorsville\tVT\tWindsor County\tH1\n5062\t50027\tReading\tVT\tWindsor County\tH1\n5060\t50027\tRandolph\tVT\tWindsor County\tH1\n5037\t50027\tBrownsville\tVT\tWindsor County\tH1\n5070\t50027\tSouth strafford\tVT\tWindsor County\tH1\n5031\t50027\tBarnard\tVT\tWindsor County\tH1\n5091\t50027\tWoodstock\tVT\tWindsor County\tH1\n5151\t50027\tPerkinsville\tVT\tWindsor County\tH1\n5067\t50027\tSouth pomfret\tVT\tWindsor County\tH1\n5065\t50027\tSharon\tVT\tWindsor County\tH1\n5068\t50027\tSouth royalton\tVT\tWindsor County\tH1\n5758\t50027\tMount holly\tVT\tWindsor County\tH1\n5772\t50027\tStockbridge\tVT\tWindsor County\tH1\n5034\t50027\tBridgewater\tVT\tWindsor County\tH1\n5049\t50027\tHartland four corners\tVT\tWindsor County\tH1\n5048\t50027\tHartland\tVT\tWindsor County\tH1\n5767\t50027\tRochester\tVT\tWindsor County\tH1\n5035\t50027\tBridgewater corners\tVT\tWindsor County\tH1\n5053\t50027\tNorth pomfret\tVT\tWindsor County\tH1\n5056\t50027\tPlymouth\tVT\tWindsor County\tH1\n5071\t50027\tSouth woodstock\tVT\tWindsor County\tH1\n5084\t50027\tWest hartford\tVT\tWindsor County\tH1\n5001\t50027\tWhite river junction\tVT\tWindsor County\tH1\n5156\t50027\tSpringfield\tVT\tWindsor County\tH1\n5161\t50027\tWeston\tVT\tWindsor County\tH1\n5075\t50027\tThetford center\tVT\tWindsor County\tH1\n5088\t50027\tWilder\tVT\tWindsor County\tH1\n5009\t50027\tWhite river junction\tVT\tWindsor County\tH1\n23301\t51001\tAccomac\tVA\tAccomack County\tH1\n23420\t51001\tPainter\tVA\tAccomack County\tH1\n23417\t51001\tOnancock\tVA\tAccomack County\tH1\n23359\t51001\tHallwood\tVA\tAccomack County\tH1\n23488\t51001\tWithams\tVA\tAccomack County\tH1\n23308\t51001\tBloxom\tVA\tAccomack County\tH1\n23356\t51001\tGreenbackville\tVA\tAccomack County\tH1\n23303\t51001\tAtlantic\tVA\tAccomack County\tH1\n23415\t51001\tNew church\tVA\tAccomack County\tH1\n23409\t51001\tMears\tVA\tAccomack County\tH1\n23404\t51001\tLocustville\tVA\tAccomack County\tH1\n23426\t51001\tSanford\tVA\tAccomack County\tH1\n23414\t51001\tNelsonia\tVA\tAccomack County\tH1\n23350\t51001\tExmore\tVA\tAccomack County\tH1\n23410\t51001\tMelfa\tVA\tAccomack County\tH1\n23422\t51001\tPungoteague\tVA\tAccomack County\tH1\n23421\t51001\tParksley\tVA\tAccomack County\tH1\n23337\t51001\tWallops island\tVA\tAccomack County\tH1\n23306\t51001\tBelle haven\tVA\tAccomack County\tH1\n23357\t51001\tGreenbush\tVA\tAccomack County\tH1\n23480\t51001\tWachapreague\tVA\tAccomack County\tH1\n23427\t51001\tSaxis\tVA\tAccomack County\tH1\n23418\t51001\tOnley\tVA\tAccomack County\tH1\n23395\t51001\tHorntown\tVA\tAccomack County\tH1\n23423\t51001\tQuinby\tVA\tAccomack County\tH1\n23416\t51001\tOak hall\tVA\tAccomack County\tH1\n23407\t51001\tMappsville\tVA\tAccomack County\tH1\n23401\t51001\tKeller\tVA\tAccomack County\tH1\n23389\t51001\tHarborton\tVA\tAccomack County\tH1\n23440\t51001\tTangier\tVA\tAccomack County\tH1\n23336\t51001\tChincoteague island\tVA\tAccomack County\tH1\n23442\t51001\tTemperanceville\tVA\tAccomack County\tH1\n23302\t51001\tAssawoman\tVA\tAccomack County\tH1\n23358\t51001\tHacksneck\tVA\tAccomack County\tH1\n23441\t51001\tTasley\tVA\tAccomack County\tH1\n23341\t51001\tCraddockville\tVA\tAccomack County\tH1\n22911\t51003\tCharlottesville\tVA\tAlbemarle County\tH1\n22920\t51003\tAfton\tVA\tAlbemarle County\tH1\n22938\t51003\tFaber\tVA\tAlbemarle County\tH1\n22932\t51003\tCrozet\tVA\tAlbemarle County\tH1\n22935\t51003\tDyke\tVA\tAlbemarle County\tH1\n22942\t51003\tGordonsville\tVA\tAlbemarle County\tH1\n22903\t51003\tCharlottesville\tVA\tAlbemarle County\tH1\n22940\t51003\tFree union\tVA\tAlbemarle County\tH1\n22943\t51003\tGreenwood\tVA\tAlbemarle County\tH1\n22909\t51003\tCharlottesville\tVA\tAlbemarle County\tH1\n22901\t51003\tCharlottesville\tVA\tAlbemarle County\tH1\n22923\t51003\tBarboursville\tVA\tAlbemarle County\tH1\n22947\t51003\tKeswick\tVA\tAlbemarle County\tH1\n22904\t51003\tCharlottesville\tVA\tAlbemarle County\tH1\n22945\t51003\tIvy\tVA\tAlbemarle County\tH1\n22902\t51003\tCharlottesville\tVA\tAlbemarle County\tH1\n22936\t51003\tEarlysville\tVA\tAlbemarle County\tH1\n22968\t51003\tRuckersville\tVA\tAlbemarle County\tH1\n22946\t51003\tKeene\tVA\tAlbemarle County\tH1\n22908\t51003\tCharlottesville\tVA\tAlbemarle County\tH1\n24562\t51003\tHowardsville\tVA\tAlbemarle County\tH1\n22959\t51003\tNorth garden\tVA\tAlbemarle County\tH1\n22987\t51003\tWhite hall\tVA\tAlbemarle County\tH1\n22937\t51003\tEsmont\tVA\tAlbemarle County\tH1\n22931\t51003\tCovesville\tVA\tAlbemarle County\tH1\n22974\t51003\tTroy\tVA\tAlbemarle County\tH1\n22969\t51003\tSchuyler\tVA\tAlbemarle County\tH1\n24590\t51003\tScottsville\tVA\tAlbemarle County\tH1\n22924\t51003\tBatesville\tVA\tAlbemarle County\tH1\n24457\t51005\tLow moor\tVA\tAlleghany County\tH1\n24085\t51005\tEagle rock\tVA\tAlleghany County\tH1\n24422\t51005\tClifton forge\tVA\tAlleghany County\tH1\n24127\t51005\tNew castle\tVA\tAlleghany County\tH1\n24448\t51005\tIron gate\tVA\tAlleghany County\tH1\n24474\t51005\tSelma\tVA\tAlleghany County\tH1\n24445\t51005\tHot springs\tVA\tAlleghany County\tH1\n24426\t51005\tCovington\tVA\tAlleghany County\tH1\n23083\t51007\tJetersville\tVA\tAmelia County\tH1\n23833\t51007\tChurch road\tVA\tAmelia County\tH1\n23966\t51007\tRice\tVA\tAmelia County\tH1\n23105\t51007\tMannboro\tVA\tAmelia County\tH1\n23002\t51007\tAmelia court house\tVA\tAmelia County\tH1\n23824\t51007\tBlackstone\tVA\tAmelia County\tH1\n23850\t51007\tFord\tVA\tAmelia County\tH1\n22967\t51009\tRoseland\tVA\tAmherst County\tH1\n22976\t51009\tTyro\tVA\tAmherst County\tH1\n24572\t51009\tMadison heights\tVA\tAmherst County\tH1\n24483\t51009\tVesuvius\tVA\tAmherst County\tH1\n22922\t51009\tArrington\tVA\tAmherst County\tH1\n24521\t51009\tAmherst\tVA\tAmherst County\tH1\n24574\t51009\tMonroe\tVA\tAmherst County\tH1\n24595\t51009\tSweet briar\tVA\tAmherst County\tH1\n24533\t51009\tClifford\tVA\tAmherst County\tH1\n24553\t51009\tGladstone\tVA\tAmherst County\tH1\n24526\t51009\tBig island\tVA\tAmherst County\tH1\n24504\t51011\tLynchburg\tVA\tAppomattox County\tH1\n24593\t51011\tSpout spring\tVA\tAppomattox County\tH1\n24538\t51011\tConcord\tVA\tAppomattox County\tH1\n23960\t51011\tProspect\tVA\tAppomattox County\tH1\n23939\t51011\tEvergreen\tVA\tAppomattox County\tH1\n24522\t51011\tAppomattox\tVA\tAppomattox County\tH1\n23958\t51011\tPamplin\tVA\tAppomattox County\tH1\n23963\t51011\tRed house\tVA\tAppomattox County\tH1\n24553\t51011\tGladstone\t
